vi "test-SequentialFileName.vi"() -> (0 "Result":errorcluster[](array[cluster]))   [LabVIEW 2021]
panel:
  out "Status":bool
  in  "String":string="# 連番部分を1増やすのが基本動作\ntest0000.dat\ntest0000.dat\ntest0001.dat\n\n# 連番部分を1増やすのが基本動作\ntest0309.dat\ntest0309.dat\ntest0310.dat\n\n# 桁数は自動的に増える\ntest99.dat\ntest99.dat\ntest100.dat\n\n# 連番がなければ勝手につける\ntest.dat\ntest0000.dat\ntest0001.dat\n\n# 拡張子も勝手につける(付けないことも可能)\ntest0000\ntest0000.dat\ntest0001.dat\n\n# 連番と拡張子両方を追加\ntest\ntest0000.dat\ntest0001.dat\n\n# もちろんパスが付いていてもOK\nC:\\path\\to\\the\\file\\test\nC:\\path\\to\\the\\file\\test0000.dat\nC:\\path\\to\\the\\file\\test0001.dat\n"
  # "テストスクリプトは\n# から始まるコメントと\n空行とを除いて\n３行ずつがセットになっている\n\n1行目が入力文字列\n2行目が連番追加後の期待値\n3行目がインクリメント後の期待値\n\nエラーの詳細は test-runner.vi で見て"
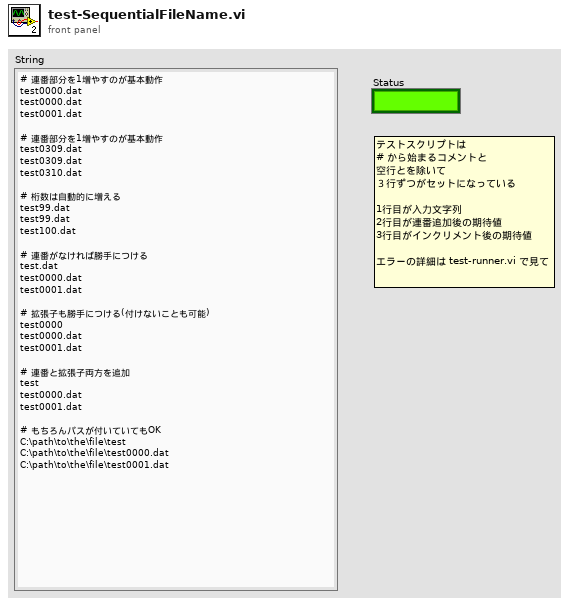
[diagram p1: front panel]
types:
  T1 = cluster{"[0]":string, "[1]":string, "[2]":string}
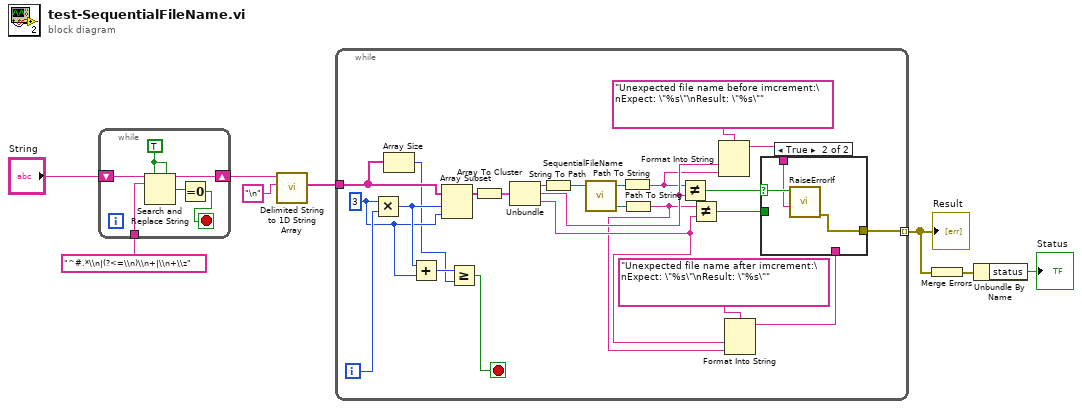
[diagram p0: block diagram]
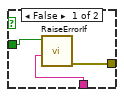
[diagram p2: hidden frame]
diagram:
  n1 = while {
    tunnel: "^#.*\\n|(?<=\\n)\\n+|\\n+\\z" ("search string") -> [w13]
    shift-right: [w11] -> w5
    shift-left: "String" -> [w14]
    stop <- w10 stop-if-true
    w12 = TRUE ("replace all? (F)")
    n2 = Search and Replace String(replace all?=w12, multiline?=w12, input string=w14, search string=w13) -> (result string=w11:string, number of replacements=w9:i32)  [unwired: 4 in, 2 out]
    n3 = Equal To 0?(x=w9) -> (x = 0?=w10:bool)
  }
  n4 = call <vilib>:"Delimited String to 1D String Array.vi"("delimiter"="\n", "delimited string"=w5) -> ("string array"=w6:string[])  [unwired: 9 in]
  n5 = while {
    tunnel: w6 -> [w18]
    tunnel: [w21] -> w3 mode=indexing
    i -> [w38]
    stop <- w15 stop-if-true
    w19 = 3 ("x")
    n6 = Multiply(x=w19, y=w38) -> (x*y=w20:i32)
    n7 = Array Size(array=w18) -> (size(s)=w16:i32)
    n8 = Add(x=w20, y=w19) -> (x+y=w17:i32)
    n9 = Array Subset(array=w18, index=w20, length=w19) -> (w37:string[])
    n10 = Greater Or Equal?(x=w17, y=w16) -> (x >= y?=w15:bool)
    n11 = Array To Cluster(array=w37) -> (cluster=w36:T1)
    n12 = Unbundle(w36) -> ("[0]"=w35:string, "[1]"=w31:string, "[2]"=w26:string)
    n13 = String To Path(string=w35) -> (path=w34:path)
    n14 = call "SequentialFileName.vi"("File Name In"=w34) -> ("Next File Name"=w32:path, "File Name With Sequence"=w33:path)  [unwired: 3 in]
    n15 = Path To String(path=w33) -> (string=w30:string)
    n16 = Path To String(path=w32) -> (string=w25:string)
    n17 = Not Equal?(x=w30, y=w31) -> (x != y?=w29:bool)
    n18 = Not Equal?(x=w25, y=w26) -> (x != y?=w23:bool)
    n19 = Format Into String(format string="Unexpected file name before imcrement:\nExpect: \"%s\"\nResult: \"%s\"", w31, w30) -> (resulting string=w24:string)  [unwired: 2 in, 1 out]
    n20 = Format Into String(format string="Unexpected file name after imcrement:\nExpect: \"%s\"\nResult: \"%s\"", w26, w25) -> (resulting string=w22:string)  [unwired: 2 in, 1 out]
    n21 = case shown="True" w29 {
      selector: w29 -> [_ w44]
      tunnel: w24 -> [_ w43]
      tunnel: w23 -> [w41 _]
      tunnel: w22 -> [w40 _]
      tunnel: [w39 w42] -> w21
      frame False {
        n22 = call "RaiseErrorIf.vi"("error message"=w40, "error? (true)"=w41) -> ("error out"=w39:errorcluster)  [unwired: 9 in]
      }
      frame True {
        n23 = call "RaiseErrorIf.vi"("error message"=w43, "error? (true)"=w44) -> ("error out"=w42:errorcluster)  [unwired: 9 in]
      }
    }
  }
  "Result" <- w3
  n24 = Merge Errors(w3) -> (w2:errorcluster)
  n25 = Unbundle By Name(w2) -> ("status"=→"Status":bool)
